vi "Reopen VISA.vi"(0 "VISA resource name":refnum<visa-resource-name>, 5 "IP Address Changed (F)?":bool, 7 "IP Address (000.000.000.000)":string="000.000.000.000", 11 "error in (no error)":errorcluster) -> (4 "VISA resource name out":refnum<visa-resource-name>, 15 "error out":errorcluster)   [LabVIEW 2020]
doc: "Reads the response from the instrument, when it is connected in serial mode (This is because the instrument sends the ACK or NACK automatically in this mode of communication)\n\nThis is a Private type VI and meant for getting the acknowledgement alone."
uses:
  Instance           2 19Saved   Reopen VISA .vi
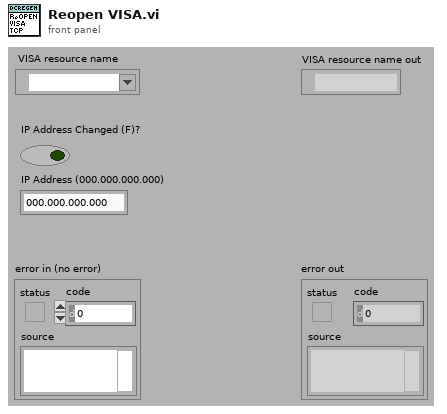
[diagram p1: front panel]
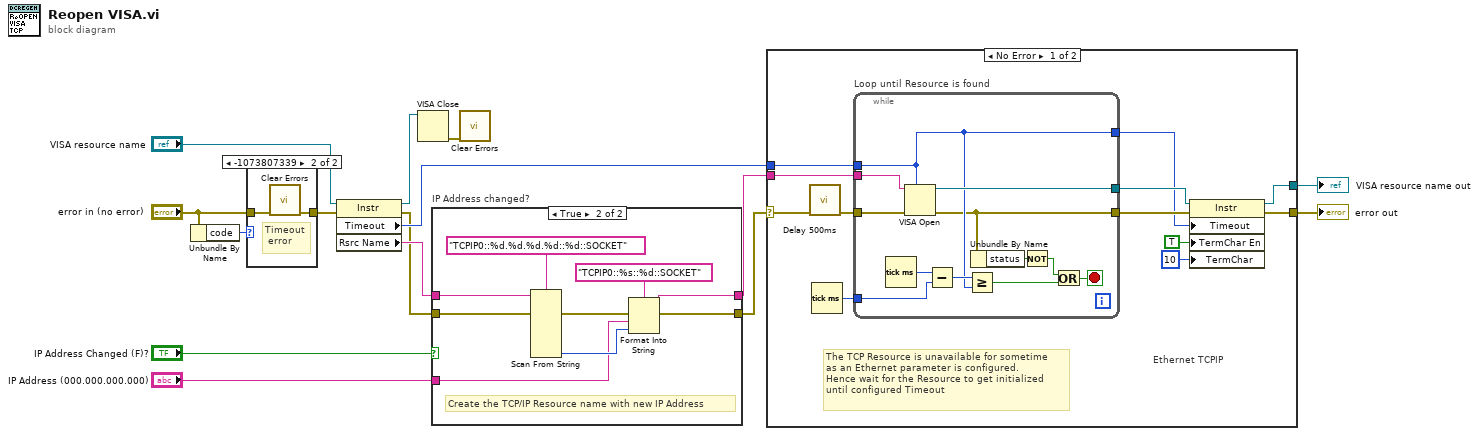
[diagram p0: block diagram]
diagram:
  n1 = Unbundle By Name("error in (no error)") -> ("code"=w12:i32)
  n2 = case shown="-1073807339" w12 {
    tunnel: "error in (no error)" -> [w16 w18]
    tunnel: [w16 w17] -> w4
    frame Default {
    }
    frame -1073807339 {
      # "Timeout\n error"
      n3 = call <vilib>:"Clear Errors.vi"("error in (no error)"=w18) -> ("error out"=w17:errorcluster)  [unwired: 5 in, 1 out]
    }
  }
  n4 = property on="Property Node" class="Instr"(reference="VISA resource name", error in=w4) -> (reference out=w7:refnum<visa-resource-name>, error out=w3:errorcluster, "Timeout"=w10:u32, "Rsrc Name"=w9:string)
  n5 = VISA Close(VISA resource name=w7) -> (error out=w1:errorcluster)  [unwired: 1 in]
  n6 = case "IP Address changed?" shown="True" "IP Address Changed (F)?" {
    tunnel: w9 -> [w20 w25]
    tunnel: "IP Address (000.000.000.000)" -> [_ w24]
    tunnel: [w20 w23] -> w6
    tunnel: w3 -> [w19 w22]
    tunnel: [w19 w21] -> w2
    frame False {
    }
    frame True {
      # "Create the TCP/IP Resource name with new IP Address"
      n7 = Scan From String(format string="TCPIP0::%d.%d.%d.%d::%d::SOCKET", input string=w25, error in=w22) -> (error out=w29:errorcluster, output 5=w26:i32)  [unwired: 10 in, 2 out]
      n8 = Format Into String(format string="TCPIP0::%s::%d::SOCKET", error in=w29, w24, w26) -> (resulting string=w23:string, error out=w21:errorcluster)  [unwired: 1 in]
    }
  }
  n9 = call <vilib>:"Clear Errors.vi"("error in (no error)"=w1) -> ()  [unwired: 5 in, 2 out]
  n10 = case shown="No Error" w2 {
    selector: w2 -> [w34 w55]
    tunnel: w6 -> [w33 w54]
    tunnel: [w39 w55] -> w15
    tunnel: [w38 w54] -> w14
    tunnel: w10 -> [w32 _]
    frame No Error {
      # "The TCP Resource is unavailable for sometime\nas an Ethernet parameter is configured.\nHence wait for the Resource to get initialized\nuntil configured Timeout"
      # "Ethernet TCPIP"
      n11 = call "Delay 500ms"("error in (no error)"=w34) -> ("error out"=w35:errorcluster)  [unwired: 10 in]
      n12 = Tick Count (ms)() -> (millisecond timer value=w37:u32)
      n13 = while "Loop until Resource is found" {
        tunnel: [w42] -> w41
        tunnel: [w45] -> w40
        tunnel: w33 -> [w53]
        tunnel: w35 -> [w52]
        tunnel: w37 -> [w50]
        tunnel: [w43] -> w36
        tunnel: w32 -> [w43]
        stop <- w46 stop-if-true
        n14 = Tick Count (ms)() -> (millisecond timer value=w51:u32)
        n15 = VISA Open(timeout (0)=w43, error in (no error)=w52, VISA resource name=w53) -> (VISA resource name=w45:refnum<visa-resource-name>, error out=w42:errorcluster)  [unwired: 2 in]
        n16 = Subtract(x=w51, y=w50) -> (x-y=w44:u32)
        n17 = Greater Or Equal?(x=w44, y=w43) -> (x >= y?=w47:bool)
        n18 = Unbundle By Name(w42) -> ("status"=w49:bool)
        n19 = Not(x=w49) -> (.not. x?=w48:bool)
        n20 = Or(x=w48, y=w47) -> (x .or. y?=w46:bool)
      }
      n21 = property on="Property Node" class="Instr"(reference=w40, error in=w41, "Timeout"=w36, "TermChar En"=TRUE ("Message Based Settings:Termination Character Enable"), "TermChar"=u8 10 ("Message Based Settings:Termination Character")) -> (reference out=w38:refnum<visa-resource-name>, error out=w39:errorcluster)
    }
    frame Error {
    }
  }
  "VISA resource name out" <- w14
  "error out" <- w15
